vi "pp_trialTypes_isValid.vi"(0 "Trial Types":T1(array[cluster]) {"Stim P2" min=0.0; "Trial Weight" step=1; "Stim P1" min=0.0; "Stim Dur (s)" min=0.0; "Trial Code" min=1 step=1}, 1 "Throw Error":bool=TRUE, 5 "Total Trials":i32=60 min=2 step=2, 11 "error in (no error)":errorcluster) -> (3 "Trial Replication Factor":i32, 4 "Paradigm Valid?":bool=TRUE, 6 "GO Trials":T1(array[cluster]) {"Stim P2" min=0.0; "Trial Weight" step=1; "Stim P1" min=0.0; "Stim Dur (s)" min=0.0; "Trial Code" min=1 step=1}, 8 "NOGO Trials":T1(array[cluster]) {"Stim P2" min=0.0; "Trial Weight" step=1; "Stim P1" min=0.0; "Stim Dur (s)" min=0.0; "Trial Code" min=1 step=1}, 10 "TEST Trials":T1(array[cluster]) {"Stim P2" min=0.0; "Trial Weight" step=1; "Stim P1" min=0.0; "Stim Dur (s)" min=0.0; "Trial Code" min=1 step=1}, 15 "error out":errorcluster)   [LabVIEW 2013]
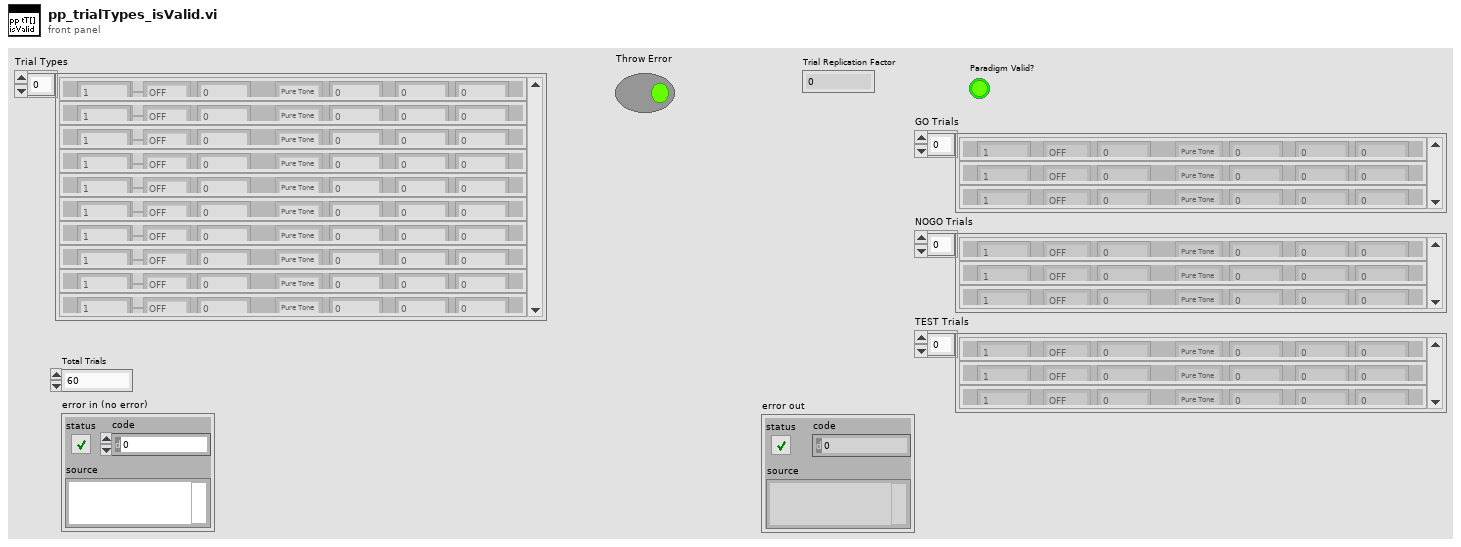
[diagram p1: front panel]
types:
  T1 = cluster{"Trial Code":u16, "Trial Type":enum16{"OFF", "GO", "NOGO", "TEST"}, "Trial Weight":u32, "Stim Type":enum16{"Pure Tone", "FM Sweep"}, "Stim Dur (s)":dbl, "Stim P1":dbl, "Stim P2":dbl}[]
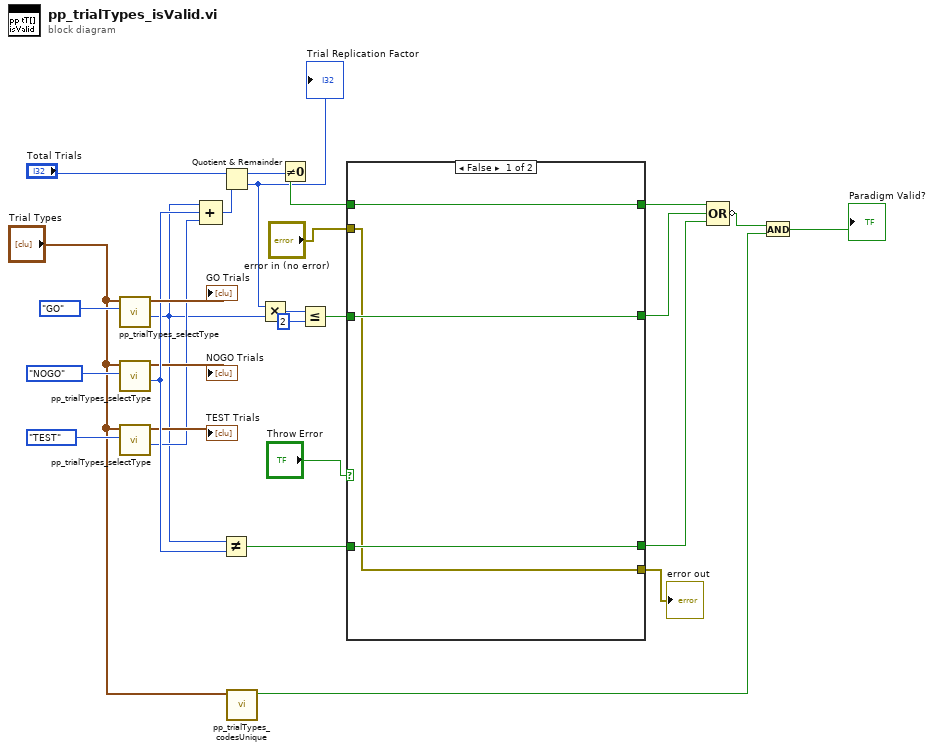
[diagram p0: block diagram]
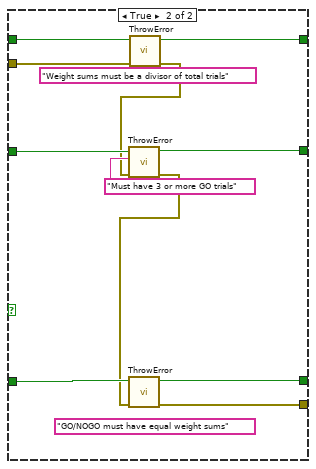
[diagram p2: hidden frame]
diagram:
  n1 = call "pp_trialTypes_selectType.vi"("Trial Type"=enum16{"OFF", "GO", "NOGO", "TEST"}."GO", "Trial Types"="Trial Types") -> ("Weight sums"=w1:i32, "Selected Trial Types"=→"GO Trials":T1)  [unwired: 7 in, 1 out]
  n2 = call "pp_trialTypes_selectType.vi"("Trial Type"=enum16{"OFF", "GO", "NOGO", "TEST"}."NOGO", "Trial Types"="Trial Types") -> ("Weight sums"=w21:i32, "Selected Trial Types"=→"NOGO Trials":T1)  [unwired: 7 in, 1 out]
  n3 = call "pp_trialTypes_selectType.vi"("Trial Type"=enum16{"OFF", "GO", "NOGO", "TEST"}."TEST", "Trial Types"="Trial Types") -> ("Weight sums"=w2:i32, "Selected Trial Types"=→"TEST Trials":T1)  [unwired: 7 in, 1 out]
  n4 = Compound Arithmetic op=ADD(w1, w21, w2) -> (w20:i32)
  n5 = Not Equal?(x=w1, y=w21) -> (x != y?=w23:bool)
  n6 = Quotient & Remainder(x="Total Trials", y=w20) -> (x-y*floor(x/y)=w5:i32, floor(x/y)=w3:i32)
  "Trial Replication Factor" <- w3
  n7 = call "pp_trialTypes_codesUnique.vi"("Trial Types"="Trial Types") -> ("Codes unique?"=w6:bool)  [unwired: 9 in, 1 out]
  n8 = Multiply(x=w3, y=w1) -> (x*y=w4:i32)
  n9 = Not Equal To 0?(x=w5) -> (x != 0?=w19:bool)
  n10 = Less Or Equal?(x=w4, y=2) -> (x <= y?=w24:bool)
  n11 = case shown="False" "Throw Error" {
    tunnel: w24 -> [w31 w43]
    tunnel: w23 -> [w30 w41]
    tunnel: w19 -> [w32 w40]
    tunnel: [w32 w37] -> w14
    tunnel: [w31 w36] -> w13
    tunnel: [w30 w35] -> w12
    tunnel: [w29 w34] -> w9
    tunnel: "error in (no error)" -> [w29 w33]
    frame False {
    }
    frame True {
      (unwired) "Weight sums must be a divisor of total trials" ("Error Message")
      (unwired) "GO/NOGO must have equal weight sums" ("Error Message")
      n12 = call "ThrowError.vi"("error in (no error)"=w33, "Error Input"=w40) -> ("error out"=w39:errorcluster, "Error Input Passthrough"=w37:bool)  [unwired: 8 in]
      n13 = call "ThrowError.vi"("error in (no error)"=w39, "Error Message"="Must have 3 or more GO trials", "Error Input"=w43) -> ("error out"=w38:errorcluster, "Error Input Passthrough"=w36:bool)  [unwired: 7 in]
      n14 = call "ThrowError.vi"("error in (no error)"=w38, "Error Input"=w41) -> ("error out"=w34:errorcluster, "Error Input Passthrough"=w35:bool)  [unwired: 8 in]
    }
  }
  "error out" <- w9
  n15 = Compound Arithmetic op=OR(w14, w13, w12) -> (invert w10:bool)
  n16 = And(x=w10, y=w6) -> (x .and. y?=→"Paradigm Valid?":bool)
